vi "Encode YAML.vi"() -> ()   [LabVIEW 2015]
uses:
  Components/YAML Parser.lvlib
panel:
  in  "Weight":dbl=80.0
  out "YAML String":string
  in  "Phones":string[](array[string])=["06.43.94.98.85", "06.43.94.98.86"]
  in  "Size":dbl=182.1
  in  "Male":bool=TRUE
  in  "Age":u32=27
  in  "Address":string="10 rue Jean Prévost\n38000 Grenoble\nFrance"
  in  "Name":string="Nicolas Bats"
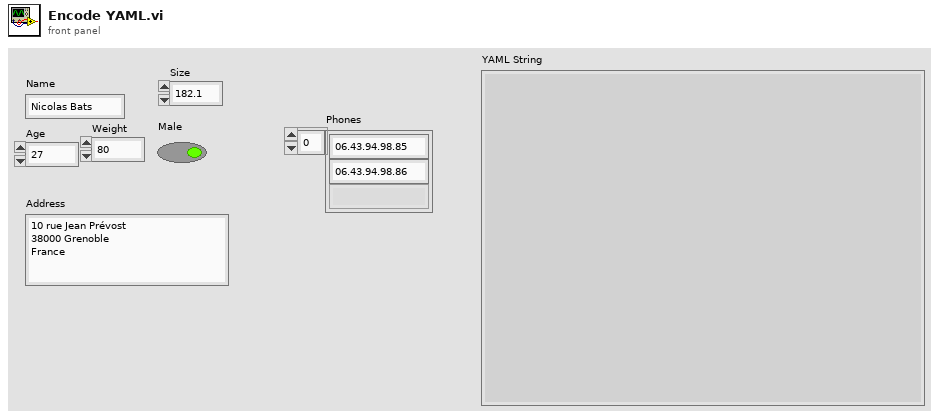
[diagram p1: front panel]
types:
  T1 = cluster{"Male":bool, "Name":string, "Age":u32, "Physical":cluster{"Size":dbl, "Weight":dbl}, "Address":string, "Phones":string[], "seconds since 1Jan1904":timestamp}
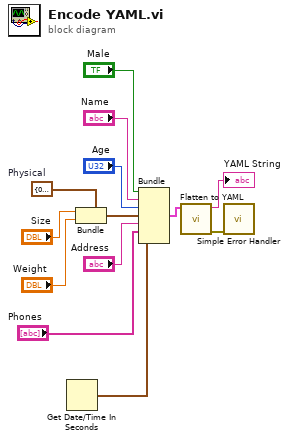
[diagram p0: block diagram]
diagram:
  w3 = cluster{"Size":dbl, "Weight":dbl} {"Size"=0.0, "Weight"=0.0}  # Physical
  n1 = Get Date/Time In Seconds() -> (seconds since 1Jan1904=w1:timestamp)
  n2 = Bundle(cluster=w3, "Size"="Size", "Weight"="Weight") -> (w4:cluster{"Size":dbl, "Weight":dbl})
  n3 = Bundle("Male"="Male", "Name"="Name", "Age"="Age", "Physical"=w4, "Address"="Address", "Phones"="Phones", "seconds since 1Jan1904"=w1) -> (w9:T1)  [unwired: 1 in]
  n4 = call "Flatten to YAML.vi"("Anything"=w9) -> ("error out"=w8:errorcluster, "YAML String"=→"YAML String":string)  [unwired: 9 in]
  n5 = call <vilib>:"Simple Error Handler.vi"("error in (no error)"=w8) -> ()  [unwired: 4 in, 5 out]
